vi "read_spectra_color_new_Flash.vi"() -> (0 "correction":dbl[](array[numeric]))   [LabVIEW 2022 SP3]
panel:
  out "Waveform Graph 2":dbl[](graph)
  out "Read_data":u8[](array[numeric])
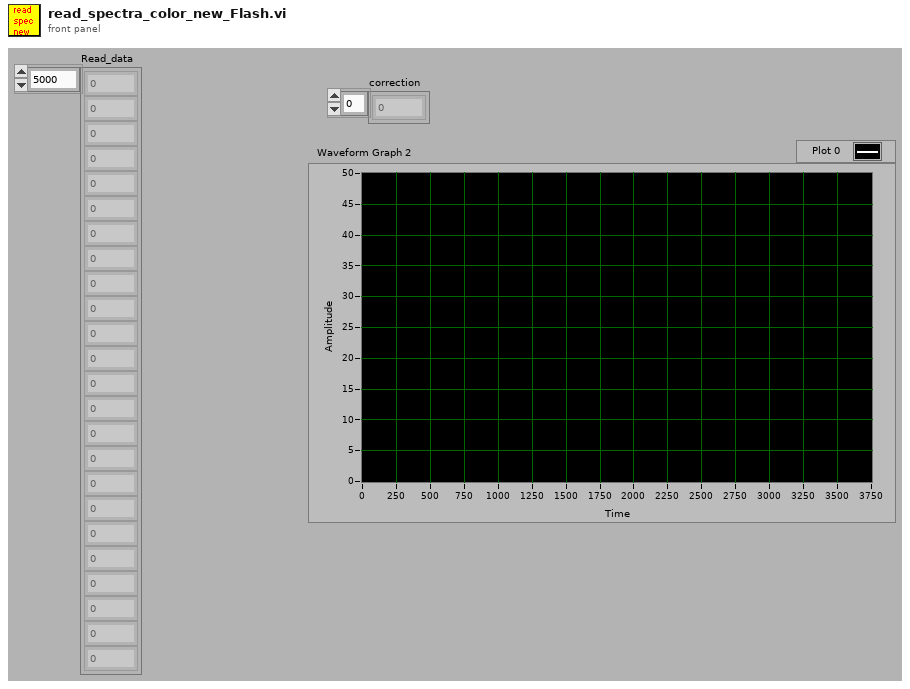
[diagram p1: front panel]
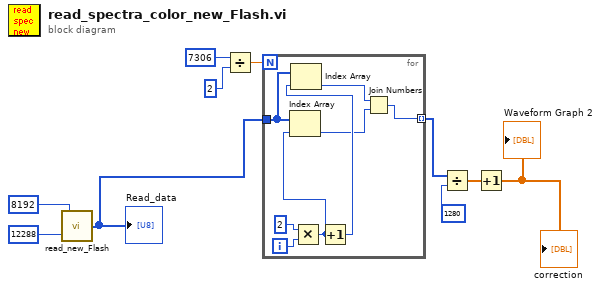
[diagram p0: block diagram]
diagram:
  n1 = call "read_new_Flash.vi"("address (3 bytes)"=u32 12288, "read_bytes"=u64 8192) -> ("Read_data"=w3:u8[])
  "Read_data" <- w3
  n2 = Divide(x=7306 ("dimension size"), y=2) -> (x/y=w8:dbl)
  n3 = for {
    N: w8 -> [_]
    tunnel: w3 -> [w15]
    tunnel: [w11] -> w4 mode=indexing
    i -> [w18]
    n4 = Multiply(x=2, y=w18) -> (x*y=w16:i32)
    n5 = Index Array(array=w15, index=w16) -> (element=w13:u8)
    n6 = Increment(x=w16) -> (x+1=w14:i32)
    n7 = Index Array(array=w15, index=w14) -> (element=w12:u8)
    n8 = Join Numbers(hi=w12, lo=w13) -> ((hi.lo)=w11:u16)
  }
  n9 = Divide(x=w4, y=u16 1280) -> (x/y=w2:dbl[])
  n10 = Increment(x=w2) -> (x+1=→"Waveform Graph 2" →"correction":dbl[])
